vi "Continuous Overflow Statistics.vi"() -> ()   [LabVIEW 2023]
doc: "Demonstrates how to use the DFD FXP Simulation VI to generate a report continuously on the performance of the quantizers in a fixed-point filter.\n\nComplete the following steps to use this VI.\n1) Run the VI.\n2) Observe the Original Signal and Filtered Signal plots in the Signals graph. Notice that they are nearly identical except for a delay.\n3) Observe the Filtering Text Report. Notice that #Operations increases continuously for all quantizers.\n4) Set the <B>Reset Statistics?</B> value to True to reset the statistics history of the simulation process. The #Operations then counts from zero."
uses:
  <vilib>/addons/Digital Filter Design/_Objects.llb/DFD Quantization Sources.ctl
  <vilib>/addons/Digital Filter Design/_Objects.llb/DFD FXP Statistics Data.ctl
  <vilib>/addons/Digital Filter Design/_Objects.llb/DFD Filter Frequence Specification (Design).ctl
  <vilib>/addons/Digital Filter Design/FXPModel.llb/DFD FXP Quantize Coef (Easy).vi
  <vilib>/Utility/VariantDataType/GetNumericFxpInfo.vi
  <vilib>/addons/Digital Filter Design/FXPSim.llb/dfd_Check Input FXP Settings.vi
  <vilib>/addons/Digital Filter Design/FXPSim.llb/dfd_Check SRate Simulation Integer Input.vi
  <vilib>/addons/Digital Filter Design/FXPSim.llb/dfd_FXP Simu.vi
  <vilib>/addons/Digital Filter Design/FXPSim.llb/SimXnode/DFD FXP Simulation.xnode
  <vilib>/addons/Digital Filter Design/_Objects.llb/DFD Filter Obj.ctl
  <vilib>/addons/Digital Filter Design/_Objects.llb/DFD Filter Coef.ctl
  <vilib>/addons/Digital Filter Design/_Objects.llb/DFD Filter Structure Type Selector.ctl
  <vilib>/addons/Digital Filter Design/_Objects.llb/dfd_Internal Quantization Settings.ctl
  <vilib>/addons/Digital Filter Design/_Objects.llb/dfd_Internal Quantization Srcs.ctl
  <vilib>/addons/Digital Filter Design/_Objects.llb/DFD Coef Norm Type.ctl
  <vilib>/ptbypt/NI_PtbyPt.lvlib
  <vilib>/addons/Digital Filter Design/NI_DigFilterLicensed.lvlib
  <vilib>/addons/Digital Filter Design/NI_DigFilter_FXP.lvlib
  <vilib>/Utility/VariantDataType/VariantType.lvlib
panel:
  in  "Reset Statistics?":bool
  out "Filtering Text Report":string
  out "Signals":cluster{"sine wave":dbl, dbl}(graph)
  in  "stop":bool
  in  "Signal Frequency [Hz]":dbl=300.0
  # "Select Help>>Show Context Help and move the cursor over the VI icon for more information."
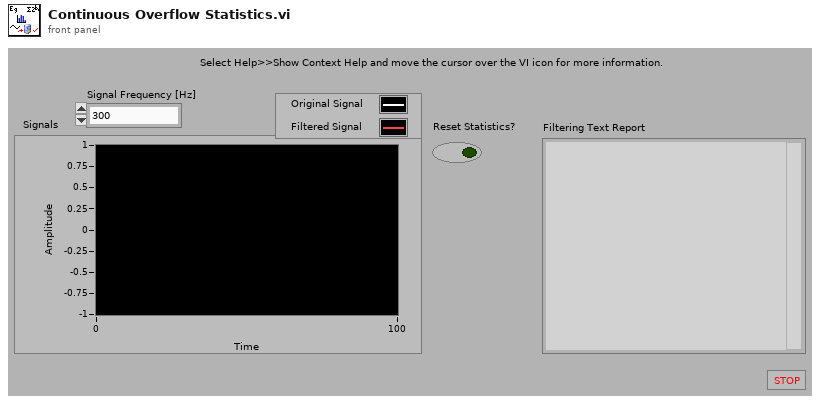
[diagram p1: front panel]
types:
  T1 = typedef "NI_DigFilterLicensed.lvlib/DFD Filter Frequence Specification (Design).ctl" = cluster{"fpass 1":dbl, "fstop 1":dbl, "fpass 2 ":dbl, "fstop 2":dbl}
  T2 = enum16{"Lowpass", "Highpass", "Bandpass", "Bandstop"}
  T3 = typedef "NI_DigFilterLicensed.lvlib/DFD Quantization Sources.ctl" = u16
  T4 = typedef "NI_DigFilterLicensed.lvlib/DFD FXP Statistics Data.ctl" = cluster{"max value":ext, "min value":ext, "#overflows":i32, "#underflows":i32, "#operations":i32}
  T5 = cluster{"Quantizer Source":T3, "statistics information":T4}[]
  T6 = typedef "NI_DigFilterLicensed.lvlib/DFD Filter Obj.ctl" = cluster{"mSRate_Fs":dbl, "mSRate_Version":string, "mSRate_Comments":string, "mSRate_OrgCoef":T7, "mSRate_CurCoef":T7, "mSRate_Quantized?":bool, "mSRate_QCoef":T7, "mSRate_QSettings":T9[], "mSRate_Order":i32, "mSRate_Scaling":cluster{"mSRate_ScaleByPowerOf2?":bool, "mSRate_ScaleType":T11}}
  T7 = typedef "NI_DigFilterLicensed.lvlib/DFD Filter Coef.ctl" = cluster{"type":T8, "gain":dbl, "coef a (k)":dbl[], "coef b (v)":dbl[]}
  T8 = typedef "NI_DigFilterLicensed.lvlib/DFD Filter Structure Type Selector.ctl" = enum16{"Undefined", "FIR Direct Form", "FIR Direct Form Transposed", "FIR Symmetric", "FIR Antisymmetric", "IIR Direct Form I", "IIR Direct Form I Transposed", "IIR Direct Form II", "IIR Direct Form II Transposed", "IIR Cascaded Second Order Sections Form I", "IIR Cascaded Second Order Sections Form I Transposed", "IIR Cascaded Second Order Sections Form II", "IIR Cascaded Second Order Sections Form II Transposed", "Lattice Allpass (basic sections)", "Lattice Allpass (one multiplier sections)", "Lattice Allpass (normalized sections)", "Lattice AR (basic sections)", "Lattice AR (one multiplier sections)", "Lattice AR (normalized sections)", "Lattice MA (minimum phase)", "Lattice MA (maximum phase)", "Lattice ARMA (basic sections)", "Lattice ARMA (one multiplier sections)", "Lattice ARMA (normalized sections)"}
  T9 = typedef "NI_DigFilterLicensed.lvlib/dfd_Internal Quantization Settings.ctl" = cluster{"source":T10, "wl":i16, "iwl":i16, "overflow mode":enum16{"Saturation", "Wrap"}, "rounding mode":enum16{"Nearest", "Truncation"}, "signed?":bool}
  T10 = typedef "NI_DigFilterLicensed.lvlib/dfd_Internal Quantization Srcs.ctl" = u16
  T11 = typedef "NI_DigFilterLicensed.lvlib/DFD Coef Norm Type.ctl" = enum16{"No Norm", "Time Domain 1-Norm", "Time Domain 2-Norm", "Time Domain Inf-Norm"}
  T12 = cluster{"quantizer source":T3, "statistics information":T4}[]
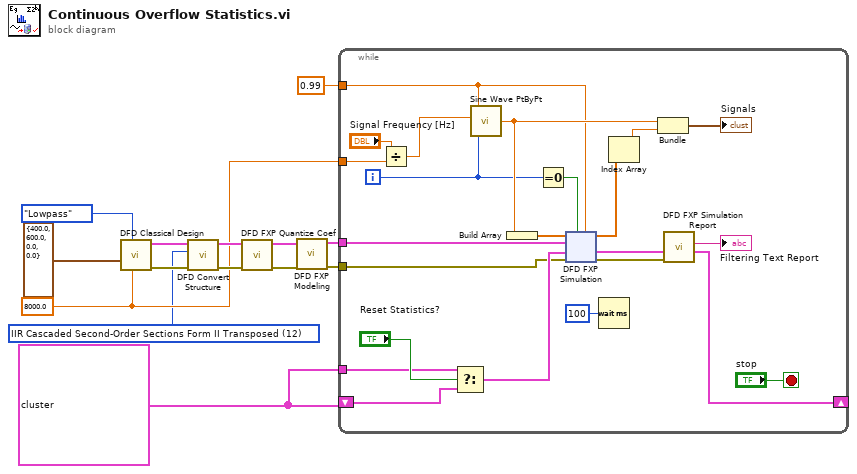
[diagram p0: block diagram]
diagram:
  w1 = u16 12 items=["FIR Direct Form"=1, "FIR Direct Form Transposed"=2, "FIR Symmetric"=3, "FIR Antisymmetric"=4, "IIR Direct Form I"=5, "IIR Direct Form I Transposed"=6, "IIR Direct Form II"=7, "IIR Direct Form II Transposed"=8, "IIR Cascaded Second-Order Sections Form I"=9, "IIR Cascaded Second-Order Sections Form I Transposed"=10, "IIR Cascaded Second-Order Sections Form II"=11, "IIR Cascaded Second-Order Sections Form II Transposed"=12, "Lattice Allpass (basic sections)"=13, "Lattice Allpass (one multiplier sections)"=14, "Lattice Allpass (normalized sections)"=15, "Lattice AR (basic sections)"=16, "Lattice AR (one multiplier sections)"=17, "Lattice AR (normalized sections)"=18, "Lattice MA (minimum phase)"=19, "Lattice MA (maximum phase)"=20, "Lattice ARMA (basic sections)"=21, "Lattice ARMA (one multiplier sections)"=22, "Lattice ARMA (normalized sections)"=23] ("target structure")
  w9 = 8000.0 ("fs [Hz]")
  w6 = T5 [{"Quantizer Source"=1, "statistics information"={"max value"=-inf, "min value"=inf, "#overflows"=0, "#underflows"=0, "#operations"=0}}, {"Quantizer Source"=2, "statistics information"={"max value"=-inf, "min value"=inf, "#overflows"=0, "#underflows"=0, "#operations"=0}}, {"Quantizer Source"=3, "statistics information"={"max value"=-inf, "min value"=inf, "#overflows"=0, "#underflows"=0, "#operations"=0}}, {"Quantizer Source"=4, "statistics information"={"max value"=-inf, "min value"=inf, "#overflows"=0, "#underflows"=0, "#operations"=0}}, {"Quantizer Source"=5, "statistics information"={"max value"=-inf, "min value"=inf, "#overflows"=0, "#underflows"=0, "#operations"=0}}, {"Quantizer Source"=6, "statistics information"={"max value"=-inf, "min value"=inf, "#overflows"=0, "#underflows"=0, "#operations"=0}}] ("filtering statistics in")
  n1 = call <vilib>:"DFD Classical Design.vi"("fs [Hz]"=w9, "filter type"=T2."Lowpass", "freq specs [Hz]"=T1 {"fpass 1"=400.0, "fstop 1"=600.0, "fpass 2 "=0.0, "fstop 2"=0.0}) -> ("error out"=w12:errorcluster, "filter out"=w13:T6)  [unwired: 4 in, 3 out]
  n2 = call <vilib>:"DFD Convert Structure.vi"("error in (no error)"=w12, "target structure"=w1, "filter in"=w13) -> ("error out"=w11:errorcluster, "filter out"=w10:T6)  [unwired: 7 out]
  n3 = call-poly <vilib>:"DFD FXP Quantize Coef.vi"("error in (no error)"=w11, "filter in"=w10) -> ("error out"=w4:errorcluster, "filter out"=w5:T6)  [unwired: 3 in, 5 out]
  n4 = call <vilib>:"DFD FXP Modeling.vi"("error in (no error)"=w4, "filter in"=w5) -> ("error out"=w2:errorcluster, "filter out"=w3:T6)  [unwired: 5 in, 3 out]
  n5 = while {
    tunnel: 0.99 ("amplitude") -> [w15]
    shift-right: [w29] -> _
    shift-left: w6 -> [w21]
    tunnel: w9 -> [w24]
    tunnel: w6 -> [w20]
    tunnel: w3 -> [w18]
    tunnel: w2 -> [w17]
    i -> [w16]
    stop <- "stop" stop-if-true
    n6 = Divide(x="Signal Frequency [Hz]", y=w24) -> (x/y=w25:dbl)
    n7 = Select(t=w20, s="Reset Statistics?", f=w21) -> (s? t:f=w19:T5)
    n8 = call <vilib>:"Sine Wave PtByPt.vi"("time"=w16, "frequency"=w25, "amplitude"=w15) -> ("sine wave"=w27:dbl)  [unwired: 1 in]
    n9 = Build Array(w27) -> (w36:dbl[])
    n10 = Equal To 0?(x=w16) -> (x = 0?=w28:bool)
    n11 = xnode "DFD FXP Simulation"("input range"=w15, "init? (T)"=w28, "error in (no error)"=w17, "filtering statistics in"=w19, "filter in"=w18, "signal in"=w36) -> ("error out"=w26:errorcluster, "filtering statistics report"=w29:T12, "DBL signal out"=w35:dbl[])  [unwired: 1 out]
    n12 = Wait (ms)(milliseconds to wait=u32 100) -> ()  [unwired: 1 out]
    n13 = Index Array(array=w35) -> (element=w34:dbl)  [unwired: 1 in]
    n14 = Bundle("sine wave"=w27, "value out"=w34) -> (→"Signals":cluster{"sine wave":dbl, "value out":dbl})  [unwired: 1 out]
    n15 = call <vilib>:"DFD FXP Simulation Report.vi"("error in (no error)"=w26, "filtering statistics report"=w29) -> ("filtering text report"=→"Filtering Text Report":string)  [unwired: 9 out]
  }
